vi "Zahvat.vi"(9 "A":bool, 10 "X":bool, 11 "Digital in":refnum<vi>) -> ()   [LabVIEW 2020]
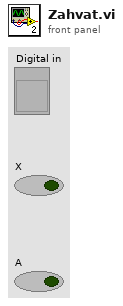
[diagram p1: front panel]
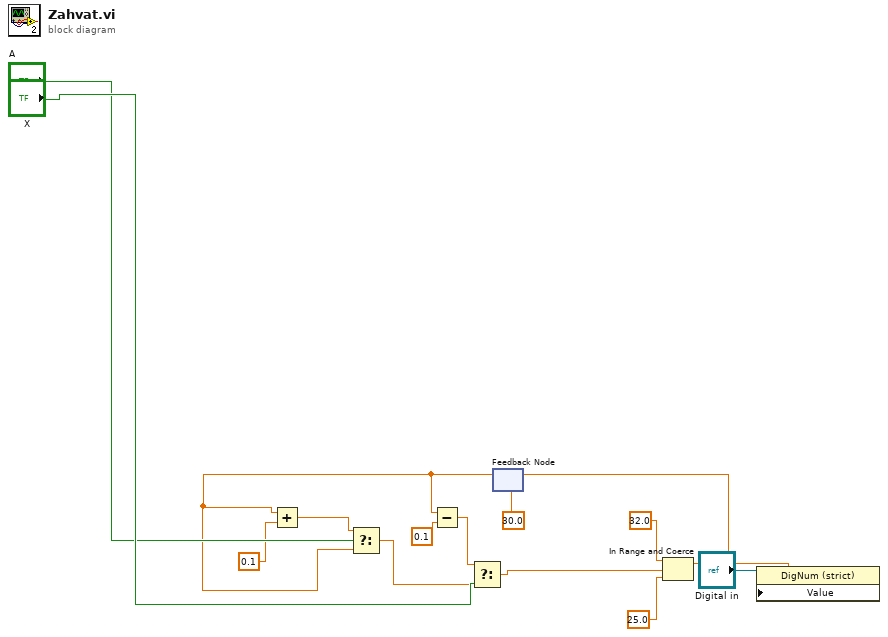
[diagram p0: block diagram]
diagram:
  n1 = feedback #1(30.0 ("upper limit")) -> (w10:dbl)
  n2 = Add(x=w10, y=0.1) -> (x+y=w5:dbl)
  n3 = Select(t=w5, s="A", f=w10) -> (s? t:f=w9:dbl)
  n4 = Subtract(x=w10, y=0.1) -> (x-y=w7:dbl)
  n5 = Select(t=w7, s="X", f=w9) -> (s? t:f=w8:dbl)
  n6 = In Range and Coerce(upper limit=32.0, x=w8, lower limit=25.0) -> (coerced(x)=w13:dbl)  [unwired: 1 out]
  n7 = feedback-in #1(w13) -> ()
  n8 = property class="DigNum (strict)"(reference="Digital in", "Value"=w13) -> ()  [unwired: 1 in, 2 out]
